vi "BMcalculate_v1_2.vi"() -> ()   [LabVIEW 2014]
uses:
  <vilib>/Analysis/coordinate.llb/2D Cartesian Coordinate Rotation (Array).vi
  <vilib>/Analysis/baseanly.llb/Mean (DBL).vi
  <vilib>/Utility/file.llb/Read From Spreadsheet File (string).vi
  <vilib>/Utility/file.llb/Write To Spreadsheet File (DBL).vi
  <vilib>/Analysis/NI_AALBase.lvlib
  <vilib>/Analysis/NI_AALPro.lvlib
panel:
  in  "Menu Ring":u16(ring) items=["No highlight", "Highlight"]
  out "created path 2":path
  out "created path":path
  in  "Save Time-trace":bool
  in  "nm/pixel":dbl=72.5 format="%#_13g"
  in  "Folder path":path
  in  "?":bool
  in  "~":dbl=1.15 format="%#_13g"
  in  "x/y for all":dbl=0.85 format="%#_13g"
  out "filename":string
  in  "Mode":u16(ring)=2 items=["Median_fix window", "Average_fix window", "Median_slide window", "Average_slide window"]
  in  "change to vertical ?":bool
  in  "?":enum32{"slide by slide", "delay"}(tab)=enum."delay"
  in  "?":bool
  in  "seconds to wait":u32
  in  "?":dbl=7.963 format="%#_13g"
  in  "?":dbl=48.61 format="%#_13g"
  in  "Save BM":bool
  in  "?":bool=TRUE
  in  "Save X-Y plot":bool
  in  "less than":dbl=0.2 format="%#_13g"
  in  "?":bool
  in  "?":bool
  in  "?":bool=TRUE
  in  "?":T1(tab)
  out "Filenames":string[](array[string])
  out "useful AOIs":i32[](array[numeric])
  out "# of AOI":i32[](array[numeric])
  out "% of useful AOIs":dbl
  out "tt # of AOIs":i32
  out "# of Frames":dbl[](array[numeric])
  out "tt # 0f useful AOIs":i32
  out "?":T2(graph)
  out "size(s)":i32
  out "X-Y plot":cluster{dbl[], dbl[]}(graph)
  out "Xstd":dbl
  out "ystd":dbl[](array[numeric])
  out "X":dbl format="%0.2f"
  out "Y":dbl format="%0.2f"
  out "?":T2(graph)
  out "tt # of useful AOIs":i32
  out "xstd":dbl[](array[numeric])
  out "# of AOI":i32
  out "y 2":dbl[](array[numeric])
  out "# of frames":dbl
  out "y":dbl[][](array[numeric])
  out "x":dbl[][](array[numeric])
  out "y":dbl[](array[numeric])
  out "x":dbl[](array[numeric])
  out "y":dbl[](array[numeric])
  out "x":dbl[](array[numeric])
  out "number":dbl[][](array[numeric])
  out "all rows":string[][](array[string])
  out "Useful aoi number":string[][](array[string])
  in  "Tab Control":enum32{"Highlight", "No Highlight"}(tab)=enum."No Highlight"
  out "Time trace HL":T3(graph)
  in  "Highlight":dbl=30.0
  in  "±":dbl=30.0
  out "aoi":string
  out "max-min":dbl
  out "Time trace":T3(graph)
  out "max-min":dbl
  out "aoi":string
  # "Critiria"
  # "±"
  # "23.776±6.613 nm"
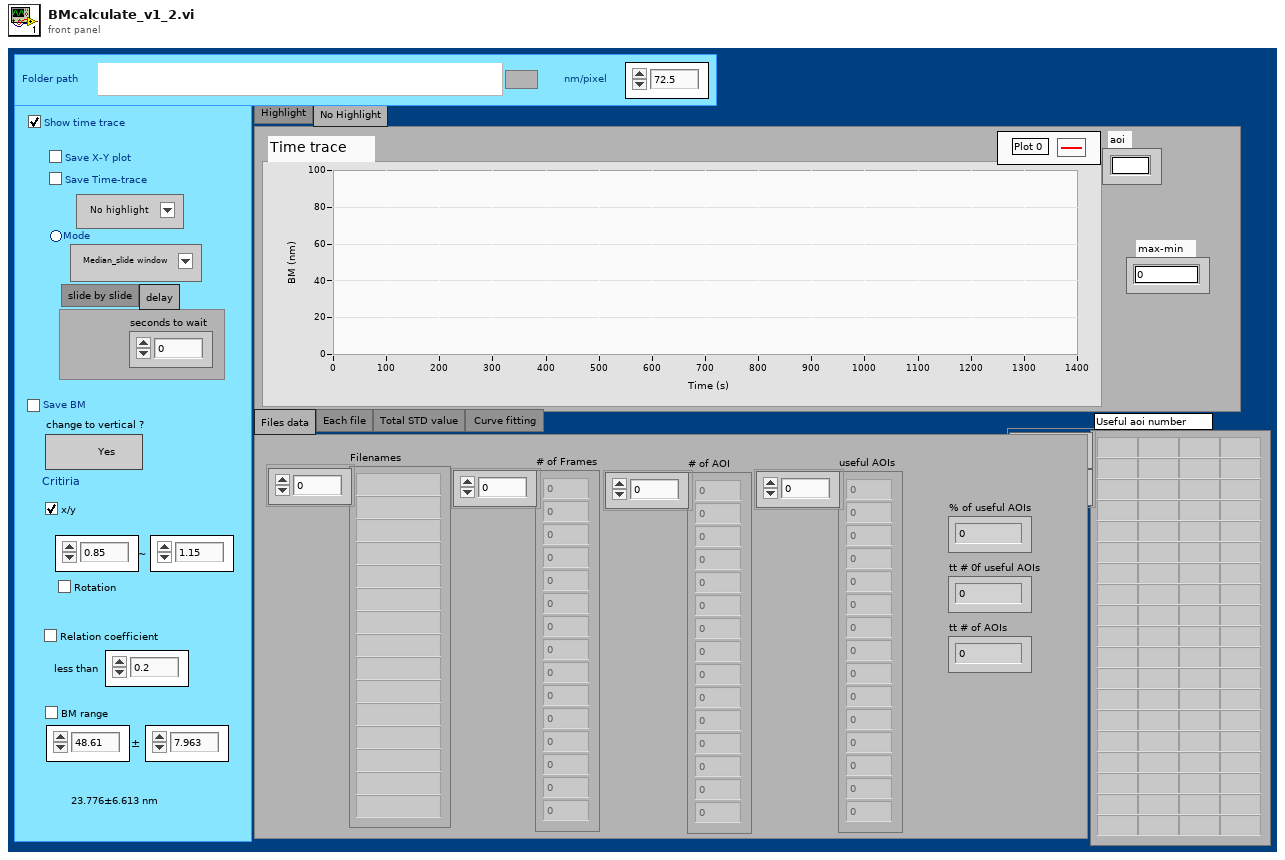
[diagram p1: front panel]
types:
  T1 = enum32{"Files data", "Each file", "Total STD value", "Curve fitting "}
  T2 = cluster{"X Values":dbl[], "Histogram: h(x)":i32[]}
  T3 = cluster{"Filtered X":dbl[], "Filtered X":dbl[]}[]
  T4 = typedef "imagedata.ctl" = cluster{"image type":i32, "image depth":i32, "image":u8[], "mask":u8[], "colors":u32[], "Rectangle":cluster{"left":i16, "top":i16, "right":i16, "bottom":i16}}
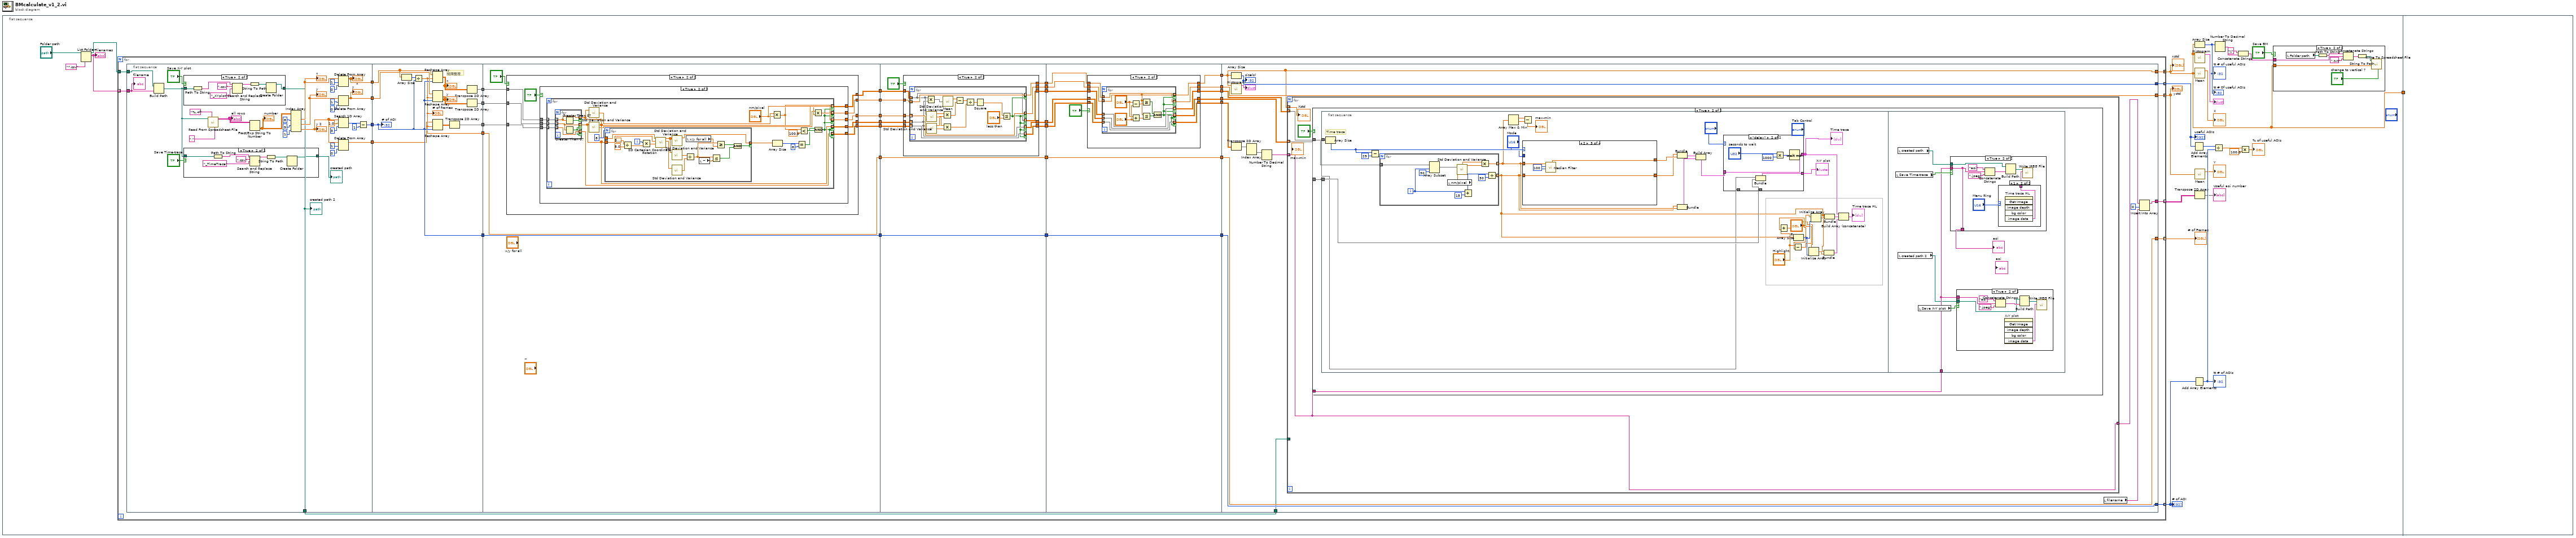
[diagram p0: block diagram]
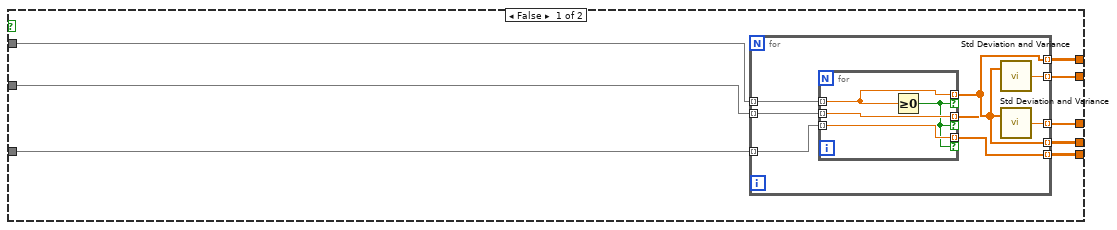
[diagram p5: hidden frame]
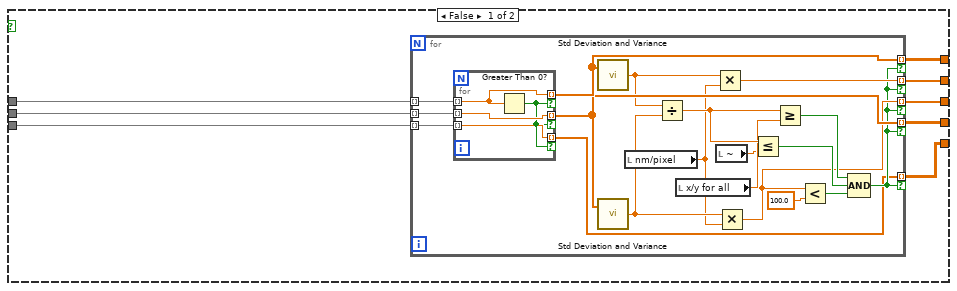
[diagram p6: hidden frame]
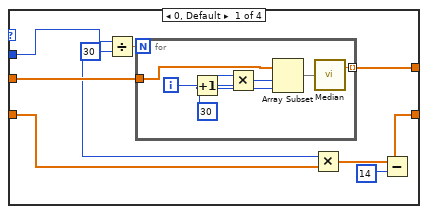
[diagram p10: hidden frame]
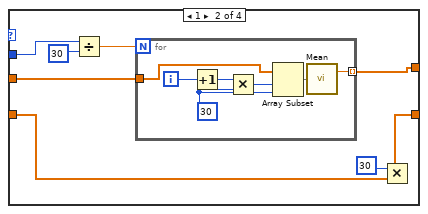
[diagram p11: hidden frame]
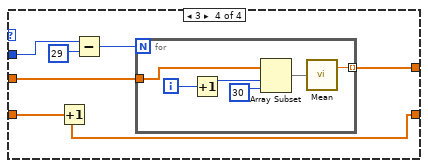
[diagram p12: hidden frame]
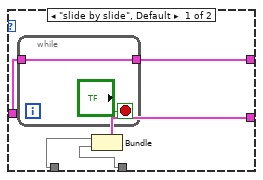
[diagram p13: hidden frame]
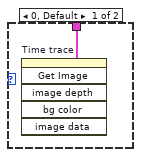
[diagram p16: hidden frame]
diagram:
  n1 = flat-sequence {
    tunnel: [w2] -> w1
    tunnel: w1 -> [_]
    frame #0 {
      n2 = List Folder(path="Folder path", pattern="*.csv") -> (path out=w24:path, filenames=w23:string[])  [unwired: 2 in, 2 out]
      "Filenames" <- w23
      n3 = for {
        tunnel: w24 -> [w37]
        tunnel: w23 -> [w72] mode=indexing
        tunnel: [w71] -> w2 mode=concatenating
        tunnel: [w70] -> w21 mode=indexing
        tunnel: [w69] -> w20 mode=indexing
        tunnel: [w68] -> w12 mode=concatenating
        tunnel: [w67] -> w13 mode=indexing
        tunnel: [w34] -> w4 mode=indexing
        n4 = flat-sequence {
          tunnel: [w92] -> w66
          tunnel: [w91] -> w65
          tunnel: [w85] -> w64
          tunnel: w37 -> [w80]
          tunnel: w72 -> [w76]
          tunnel: [w81] -> w41
          tunnel: [w79] -> w35
          tunnel: w66 -> [w128]
          tunnel: w65 -> [w127]
          tunnel: w64 -> [w124]
          tunnel: [w123] -> w63
          tunnel: [w124] -> w62
          tunnel: [w126] -> w61
          tunnel: [w125] -> w60
          tunnel: w41 -> [w122]
          tunnel: [w120] -> w40
          tunnel: w63 -> [w142]
          tunnel: w62 -> [w141]
          tunnel: w61 -> [w140]
          tunnel: w60 -> [w139]
          tunnel: [w141] -> w53
          tunnel: [w142] -> w51
          tunnel: [w137] -> w49
          tunnel: [w136] -> w47
          tunnel: [w135] -> w45
          tunnel: [w134] -> w43
          tunnel: w40 -> [w132]
          tunnel: [w133] -> w39
          tunnel: w53 -> [w265]
          tunnel: [w265] -> w52
          tunnel: w51 -> [w264]
          tunnel: [w264] -> w50
          tunnel: w49 -> [w260]
          tunnel: [w255] -> w48
          tunnel: w47 -> [w263]
          tunnel: [w258] -> w46
          tunnel: w45 -> [w262]
          tunnel: [w257] -> w44
          tunnel: w43 -> [w261]
          tunnel: [w256] -> w42
          tunnel: w39 -> [w254]
          tunnel: [w253] -> w38
          tunnel: w52 -> [w311]
          tunnel: w50 -> [w310]
          tunnel: w48 -> [w305]
          tunnel: [w311] -> w59
          tunnel: [w310] -> w58
          tunnel: [w304] -> w57
          tunnel: [w308] -> w56
          tunnel: w46 -> [w309]
          tunnel: [w306] -> w55
          tunnel: w44 -> [w307]
          tunnel: [w299] -> w54
          tunnel: w42 -> [w300]
          tunnel: w38 -> [w302]
          tunnel: [w301] -> w36
          tunnel: [w355] -> w68
          tunnel: [w356] -> w67
          tunnel: [w357] -> w69
          tunnel: [w351] -> w70
          tunnel: [w345] -> w71
          tunnel: w59 -> [w357]
          tunnel: w58 -> [w356]
          tunnel: w57 -> [w355]
          tunnel: w56 -> [w354]
          tunnel: w55 -> [w353]
          tunnel: w54 -> [w345]
          tunnel: w36 -> [w350]
          tunnel: w35 -> [w346]
          tunnel: [w341] -> w34
          frame #0 {
            n5 = Build Path(base path=w80, name or relative path=w76) -> (appended path=w74:path)
            n6 = case shown="True" "Save X-Y plot" {
              tunnel: w74 -> [w112 w119]
              tunnel: [w112 w113] -> w79
              frame False {
              }
              frame True {
                n7 = Path To String(path=w119) -> (string=w118:string)
                n8 = Search and Replace String(input string=w118, search string=".csv", replace string="_XYplot" ("replace string (\"\")")) -> (result string=w115:string)  [unwired: 5 in, 3 out]
                n9 = String To Path(string=w115) -> (path=w114:path)
                n10 = Create Folder(path (use dialog)=w114) -> (created path=w113:path)  [unwired: 2 in, 2 out]
              }
            }
            "created path 2" <- w79
            n11 = case shown="True" "Save Time-trace" {
              tunnel: w74 -> [w104 w111]
              tunnel: [w104 w105] -> w73
              frame False {
              }
              frame True {
                n12 = Path To String(path=w111) -> (string=w110:string)
                n13 = Search and Replace String(input string=w110, search string=".csv", replace string="_TimeTrace" ("replace string (\"\")")) -> (result string=w107:string)  [unwired: 5 in, 3 out]
                n14 = String To Path(string=w107) -> (path=w106:path)
                n15 = Create Folder(path (use dialog)=w106) -> (created path=w105:path)  [unwired: 2 in, 2 out]
              }
            }
            "created path" <- w73
            n16 = call-poly <vilib>:"Read From Spreadsheet File.vi"("delimiter (\\t)"="," ("delimiter (\\t)"), "format (%s)"="%.4f" ("format (%.3f)"), "file path (dialog if empty)"=w74) -> ("all rows"=w102:string[][])  [unwired: 4 in, 4 out]
            "all rows" <- w102
            n17 = Fract/Exp String To Number(string=w102) -> (number=w101:dbl[][])  [unwired: 3 in, 1 out]
            "number" <- w101
            n18 = Index Array(array=w101, index (col) #1=8 ("disabled index (col)"), index (col) #2=9 ("index (col)"), index (col) #3=1 ("index (col)")) -> (element #1=w93:dbl[], element #2=w94:dbl[], element #3=w82:dbl[])  [unwired: 3 in]
            "x" <- w93
            "y" <- w94
            "y 2" <- w82
            n19 = Delete From Array(array=w93, length=1, index=0) -> (array with subset deleted=w92:dbl[])  [unwired: 1 out]
            "x" <- w92
            n20 = Delete From Array(array=w94, length=1, index=0) -> (array with subset deleted=w91:dbl[])  [unwired: 1 out]
            "y" <- w91
            n21 = Search 1D Array(1D array=w82, element=1.0, start index (0)=3) -> (index of element=w87:i32)
            n22 = Delete From Array(array=w82, length=1, index=0) -> (array with subset deleted=w81:dbl[])  [unwired: 1 out]
            n23 = Subtract(x=w87, y=1) -> (x-y=w85:i32)
            "filename" <- w76
          }
          frame #1 {
            # "矩陣整理"
            n24 = Array Size(array=w128) -> (size(s)=w129:i32)
            n25 = Divide(x=w129, y=w124) -> (x/y=w123:dbl)
            "# of frames" <- w123
            n26 = Reshape Array(w128, w123, w124) -> (w130:dbl[][])
            "x" <- w130
            n27 = Reshape Array(w127, w123, w124) -> (w131:dbl[][])
            "y" <- w131
            n28 = Reshape Array(w122, w123, w124) -> (w121:dbl[][])
            n29 = Transpose 2D Array(2D array=w121) -> (transposed array=w120:dbl[][])
            n30 = Transpose 2D Array(2D array=w130) -> (transposed array=w126:dbl[][])
            n31 = Transpose 2D Array(2D array=w131) -> (transposed array=w125:dbl[][])
            "# of AOI" <- w124
          }
          frame #2 {
            n32 = case shown="True" "?" {
              tunnel: [w148 w171] -> w136
              tunnel: [w147 w170] -> w135
              tunnel: w140 -> [w150 w169]
              tunnel: w139 -> [w149 w168]
              tunnel: [w146 w167] -> w134
              tunnel: [w145 w166] -> w137
              tunnel: w132 -> [w144 w164]
              tunnel: [w143 w163] -> w133
              frame False {
                n33 = for {
                  tunnel: w150 -> [w158] mode=indexing
                  tunnel: w149 -> [w157] mode=indexing
                  tunnel: [w156] -> w148 mode=indexing
                  tunnel: [w155] -> w147 mode=indexing
                  tunnel: [w154] -> w146 mode=indexing
                  tunnel: [w153] -> w145 mode=indexing
                  tunnel: w144 -> [w152] mode=indexing
                  tunnel: [w151] -> w143 mode=indexing
                  n34 = for {
                    tunnel: w158 -> [w161] mode=indexing
                    tunnel: w157 -> [w162] mode=indexing
                    tunnel: [w161] -> w156 mode=indexing if=w159
                    tunnel: [w162] -> w155 mode=indexing if=w159
                    tunnel: w152 -> [w160] mode=indexing
                    tunnel: [w160] -> w151 mode=indexing if=w159
                    n35 = Greater Or Equal To 0?(x=w161) -> (x >= 0?=w159:bool)
                  }
                  n36 = call <vilib>:"Std Deviation and Variance.vi"("X"=w155) -> ("standard deviation"=w153:dbl)  [unwired: 1 in, 2 out]
                  n37 = call <vilib>:"Std Deviation and Variance.vi"("X"=w156) -> ("standard deviation"=w154:dbl)  [unwired: 1 in, 2 out]
                }
              }
              frame True {
                n38 = case shown="True" "?" {
                  tunnel: w168 -> [w178 w210]
                  tunnel: w169 -> [w179 w209]
                  tunnel: [w177 w208] -> w171
                  tunnel: [w176 w207] -> w170
                  tunnel: [w175 w206] -> w167
                  tunnel: [w174 w205] -> w166
                  tunnel: w164 -> [w173 w204]
                  tunnel: [w172 w203] -> w163
                  frame False {
                    n39 = for {
                      tunnel: w179 -> [w198] mode=indexing
                      tunnel: w178 -> [w197] mode=indexing
                      tunnel: [w196] -> w177 mode=indexing if=w183
                      tunnel: [w195] -> w176 mode=indexing if=w183
                      tunnel: [w184] -> w175 mode=indexing if=w183
                      tunnel: [w187] -> w174 mode=indexing if=w183
                      tunnel: [w181] -> w172 mode=indexing if=w183
                      tunnel: w173 -> [w182] mode=indexing
                      n40 = for {
                        tunnel: w198 -> [w201] mode=indexing
                        tunnel: w197 -> [w202] mode=indexing
                        tunnel: [w201] -> w196 mode=indexing if=w199
                        tunnel: [w202] -> w195 mode=indexing if=w199
                        tunnel: w182 -> [w200] mode=indexing
                        tunnel: [w200] -> w181 mode=indexing if=w199
                        n41 = Greater Than 0?(x=w201) -> (x > 0?=w199:bool)
                      }
                      n42 = call <vilib>:"Std Deviation and Variance.vi"("X"=w196) -> ("standard deviation"=w188:dbl)  [unwired: 1 in, 2 out]
                      n43 = call <vilib>:"Std Deviation and Variance.vi"("X"=w195) -> ("standard deviation"=w189:dbl)  [unwired: 1 in, 2 out]
                      n44 = local read "nm/pixel"() -> (w180:dbl)
                      n45 = Divide(x=w188, y=w189) -> (x/y=w194:dbl)
                      n46 = local read "x/y for all"() -> (w193:dbl)
                      n47 = Multiply(x=w188, y=w180) -> (x*y=w187:dbl)
                      n48 = local read "~"() -> (w192:dbl)
                      n49 = Multiply(x=w189, y=w180) -> (x*y=w184:dbl)
                      n50 = Less Or Equal?(x=w194, y=w192) -> (x <= y?=w190:bool)
                      n51 = Greater Or Equal?(x=w194, y=w193) -> (x >= y?=w191:bool)
                      n52 = Less?(x=w184, y=100.0) -> (x < y?=w185:bool)
                      n53 = Compound Arithmetic op=AND(w191, w190, w185) -> (w183:bool)
                    }
                  }
                  frame True {
                    n54 = for {
                      tunnel: w209 -> [w229] mode=indexing
                      tunnel: w210 -> [w228] mode=indexing
                      tunnel: [w214] -> w206 mode=indexing if=w213
                      tunnel: [w221] -> w207 mode=indexing if=w213
                      tunnel: [w222] -> w208 mode=indexing if=w213
                      tunnel: [w219] -> w205 mode=indexing if=w213
                      tunnel: [w211] -> w203 mode=indexing if=w213
                      tunnel: w204 -> [w212] mode=indexing
                      n55 = for {
                        tunnel: [w232] -> w221 mode=indexing if=w230
                        tunnel: [w233] -> w222 mode=indexing if=w234
                        tunnel: w229 -> [w233] mode=indexing
                        tunnel: w228 -> [w232] mode=indexing
                        tunnel: [w231] -> w211 mode=indexing if=w230
                        tunnel: w212 -> [w231] mode=indexing
                        n56 = Greater Than 0?(x=w233) -> (x > 0?=w234:bool)
                        n57 = Greater Than 0?(x=w232) -> (x > 0?=w230:bool)
                      }
                      n58 = call <vilib>:"Std Deviation and Variance.vi"("X"=w222) -> ("standard deviation"=w223:dbl)  [unwired: 1 in, 2 out]
                      n59 = call <vilib>:"Std Deviation and Variance.vi"("X"=w221) -> ("standard deviation"=w220:dbl)  [unwired: 1 in, 2 out]
                      n60 = for {
                        N: 8 -> [_]
                        tunnel: w222 -> [w247]
                        tunnel: w221 -> [w246]
                        tunnel: [w238] -> w224 mode=indexing if=w237
                        i -> [w248]
                        n61 = Divide(x=3.141592653589793, y=8.0) -> (x/y=w251:dbl)
                        n62 = Multiply(x=w248, y=w251) -> (x*y=w249:dbl)
                        n63 = call-poly <vilib>:"2D Cartesian Coordinate Rotation.vi"("theta"=w249, "Y"=w246, "X"=w247) -> ("Y Out"=w239:dbl[], "X Out"=w240:dbl[])  [unwired: 6 in, 1 out]
                        n64 = call <vilib>:"Std Deviation and Variance.vi"("X"=w240) -> ("mean"=w238:dbl)  [unwired: 1 in, 2 out]
                        n65 = call <vilib>:"Std Deviation and Variance.vi"("X"=w240) -> ("standard deviation"=w245:dbl)  [unwired: 1 in, 2 out]
                        n66 = call <vilib>:"Std Deviation and Variance.vi"("X"=w239) -> ("standard deviation"=w244:dbl)  [unwired: 1 in, 2 out]
                        n67 = Divide(x=w245, y=w244) -> (x/y=w243:dbl)
                        n68 = local read "x/y for all"() -> (w236:dbl)
                        n69 = local read "~"() -> (w235:dbl)
                        n70 = Less Or Equal?(x=w243, y=w235) -> (x <= y?=w241:bool)
                        n71 = Greater Or Equal?(x=w243, y=w236) -> (x >= y?=w242:bool)
                        n72 = Compound Arithmetic op=AND(w242, w241) -> (w237:bool)
                      }
                      n73 = Multiply(x=w223, y="nm/pixel") -> (x*y=w214:dbl)
                      n74 = Array Size(array=w224) -> (size(s)=w226:i32)
                      n75 = Equal?(x=w226, y=8) -> (x = y?=w215:bool)
                      n76 = Less?(x=w214, y=100.0) -> (x < y?=w216:bool)
                      n77 = Multiply(x=w220, y="nm/pixel") -> (x*y=w219:dbl)
                      n78 = Compound Arithmetic op=AND(w215, w216) -> (w213:bool)
                    }
                  }
                }
              }
            }
          }
          frame #3 {
            n79 = case shown="True" "?" {
              tunnel: w263 -> [w270 w280]
              tunnel: w262 -> [w269 w279]
              tunnel: w261 -> [w268 w276]
              tunnel: w260 -> [w267 w274]
              tunnel: [w270 w278] -> w258
              tunnel: [w269 w277] -> w257
              tunnel: [w268 w275] -> w256
              tunnel: [w267 w273] -> w255
              tunnel: w254 -> [w266 w272]
              tunnel: [w266 w271] -> w253
              frame False {
              }
              frame True {
                n80 = for {
                  tunnel: w280 -> [w286] mode=indexing
                  tunnel: w279 -> [w285] mode=indexing
                  tunnel: [w286] -> w278 mode=indexing if=w281
                  tunnel: [w285] -> w277 mode=indexing if=w281
                  tunnel: [w293] -> w275 mode=indexing if=w281
                  tunnel: w276 -> [w293] mode=indexing
                  tunnel: w274 -> [w292] mode=indexing
                  tunnel: [w292] -> w273 mode=indexing if=w281
                  tunnel: [w282] -> w271 mode=indexing if=w281
                  tunnel: w272 -> [w282] mode=indexing
                  n81 = Multiply(x=w286, y=w285) -> (x*y=w284:dbl[])
                  n82 = call <vilib>:"Std Deviation and Variance.vi"("X"=w286) -> ("mean"=w289:dbl, "standard deviation"=w291:dbl)  [unwired: 1 in, 1 out]
                  n83 = call <vilib>:"Std Deviation and Variance.vi"("X"=w285) -> ("mean"=w288:dbl, "standard deviation"=w290:dbl)  [unwired: 1 in, 1 out]
                  n84 = Multiply(x=w289, y=w288) -> (x*y=w287:dbl)
                  n85 = Multiply(x=w291, y=w290) -> (x*y=w294:dbl)
                  n86 = call-poly <vilib>:"Mean.vi"("X"=w284) -> ("mean"=w283:dbl)  [unwired: 1 out]
                  n87 = Subtract(x=w283, y=w287) -> (x-y=w295:dbl)
                  n88 = Divide(x=w295, y=w294) -> (x/y=w296:dbl)
                  n89 = Square(x=w296) -> (x^2=w297:dbl)
                  n90 = Less Or Equal?(x=w297, y="less than") -> (x <= y?=w281:bool)
                }
              }
            }
          }
          frame #4 {
            n91 = case shown="True" "?" {
              tunnel: [w317 w327] -> w308
              tunnel: w309 -> [w317 w328]
              tunnel: w307 -> [w316 w326]
              tunnel: [w316 w325] -> w306
              tunnel: w300 -> [w315 w324]
              tunnel: [w315 w323] -> w299
              tunnel: w305 -> [w314 w322]
              tunnel: [w314 w321] -> w304
              tunnel: w302 -> [w313 w320]
              tunnel: [w312 w319] -> w301
              frame False {
                n92 = for {
                  tunnel: w313 -> [w318] mode=indexing
                  tunnel: [w318] -> w312 mode=indexing
                }
              }
              frame True {
                n93 = for {
                  tunnel: [w340] -> w327 mode=indexing if=w335
                  tunnel: w328 -> [w340] mode=indexing
                  tunnel: [w339] -> w325 mode=indexing if=w335
                  tunnel: w326 -> [w339] mode=indexing
                  tunnel: [w329] -> w323 mode=indexing if=w335
                  tunnel: w324 -> [w329] mode=indexing
                  tunnel: w322 -> [w334] mode=indexing
                  tunnel: [w334] -> w321 mode=indexing if=w335
                  tunnel: [w336] -> w319 mode=indexing if=w335
                  tunnel: w320 -> [w336] mode=indexing
                  n94 = Subtract(x="?", y="?") -> (x-y=w331:dbl)
                  n95 = Add(x="?", y="?") -> (x+y=w330:dbl)
                  n96 = Greater Or Equal?(x=w329, y=w331) -> (x >= y?=w338:bool)
                  n97 = Less Or Equal?(x=w329, y=w330) -> (x <= y?=w337:bool)
                  n98 = Compound Arithmetic op=AND(w338, w337) -> (w335:bool)
                }
              }
            }
          }
          frame #5 {
            n99 = Array Size(array=w345) -> (size(s)=w351:i32)
            "size(s)" <- w351
            n100 = call <vilib>:"Histogram.vi"("X"=w345) -> ("Histogram Graph"=→"?":T2)  [unwired: 7 in, 3 out]
            n101 = Transpose 2D Array(2D array=w350) -> (transposed array=w349:dbl[][])
            n102 = Index Array(array=w349) -> (element=w348:dbl[])  [unwired: 2 in]
            n103 = Number To Decimal String(number=w348) -> (decimal integer string=w347:string[])  [unwired: 1 in]
            n104 = for {
              tunnel: w354 -> [w361] mode=indexing
              tunnel: w353 -> [w362] mode=indexing
              tunnel: w347 -> [w358] mode=indexing
              tunnel: w346 -> [_]
              tunnel: w345 -> [w359] mode=indexing
              tunnel: [w358] -> w342 mode=indexing
              n105 = case shown="True" "?" {
                tunnel: w362 -> [_ w365]
                tunnel: w361 -> [_ w364]
                tunnel: w358 -> [_ w363]
                frame False {
                }
                frame True {
                  n106 = flat-sequence {
                    tunnel: w365 -> [w378]
                    tunnel: w364 -> [w377]
                    tunnel: w363 -> [w471]
                    frame #0 {
                      # "Time trace"
                      n107 = Array Size(array=w377) -> (size(s)=w384:i32)
                      n108 = Subtract(x=w384, y=29) -> (x-y=w393:i32)
                      n109 = for {
                        N: w393 -> [_]
                        tunnel: w377 -> [w467]
                        tunnel: [w458] -> w375 mode=indexing
                        tunnel: [w460] -> w371 mode=indexing
                        i -> [w459]
                        n110 = Array Subset(array=w467, index=w459, length=30) -> (w465:dbl[])
                        n111 = local read "nm/pixel"() -> (w457:dbl)
                        n112 = call <vilib>:"Std Deviation and Variance.vi"("X"=w465) -> ("standard deviation"=w464:dbl)  [unwired: 1 in, 2 out]
                        n113 = Add(x=w459, y=15) -> (x+y=w462:i32)
                        n114 = Multiply(x=w464, y=w457) -> (x*y=w458:dbl)
                        n115 = Divide(x=w462, y=30) -> (x/y=w460:dbl)
                      }
                      n116 = Array Max & Min(array=w375) -> (max value=w390:dbl, min value=w389:dbl)  [unwired: 2 out]
                      n117 = case shown="2" "Mode" {
                        tunnel: [w402 w417 w427 w435] -> w392
                        tunnel: w375 -> [w403 w418 w428 w436]
                        tunnel: w384 -> [w401 w416 _ w434]
                        tunnel: w371 -> [w399 w412 w426 w431]
                        tunnel: [w396 w411 w426 w430] -> w376
                        frame 0, Default {
                          w397 = 30 ("y")
                          n118 = Divide(x=w401, y=w397) -> (x/y=w400:dbl)
                          n119 = for {
                            N: w400 -> [_]
                            tunnel: w403 -> [w410]
                            tunnel: [w406] -> w402 mode=indexing
                            i -> [w409]
                            w404 = 30 ("length")
                            n120 = Increment(x=w409) -> (x+1=w408:i32)
                            n121 = Multiply(x=w404, y=w408) -> (x*y=w405:i32)
                            n122 = Array Subset(array=w410, index=w405, length=w404) -> (w407:dbl[])
                            n123 = call <vilib>:"Median.vi"("X"=w407) -> ("median"=w406:dbl)  [unwired: 1 out]
                          }
                          n124 = Multiply(x=w397, y=w399) -> (x*y=w398:dbl[])
                          n125 = Subtract(x=w398, y=14) -> (x-y=w396:dbl[])
                        }
                        frame 1 {
                          n126 = Divide(x=w416, y=30) -> (x/y=w414:dbl)
                          n127 = for {
                            N: w414 -> [_]
                            tunnel: w418 -> [w425]
                            tunnel: [w422] -> w417 mode=indexing
                            i -> [w424]
                            w419 = 30 ("length")
                            n128 = Increment(x=w424) -> (x+1=w420:i32)
                            n129 = Multiply(x=w420, y=w419) -> (x*y=w421:i32)
                            n130 = Array Subset(array=w425, index=w421, length=w419) -> (w423:dbl[])
                            n131 = call-poly <vilib>:"Mean.vi"("X"=w423) -> ("mean"=w422:dbl)  [unwired: 1 out]
                          }
                          n132 = Multiply(x=30 ("length"), y=w412) -> (x*y=w411:dbl[])
                        }
                        frame 2 {
                          w429 = 100 ("left rank")
                          n133 = call <vilib>:"Median Filter.vi"("right rank"=w429, "left rank"=w429, "X"=w428) -> ("Filtered X"=w427:dbl[])  [unwired: 7 in, 1 out]
                        }
                        frame 3 {
                          n134 = Increment(x=w431) -> (x+1=w430:dbl[])
                          n135 = Subtract(x=w434, y=29) -> (x-y=w432:i32)
                          n136 = for {
                            N: w432 -> [_]
                            tunnel: w436 -> [w442]
                            tunnel: [w439] -> w435 mode=indexing
                            i -> [w441]
                            n137 = Increment(x=w441) -> (x+1=w437:i32)
                            n138 = Array Subset(array=w442, index=w437, length=30) -> (w440:dbl[])
                            n139 = call-poly <vilib>:"Mean.vi"("X"=w440) -> ("mean"=w439:dbl)  [unwired: 1 out]
                          }
                        }
                      }
                      n140 = Subtract(x=w390, y=w389) -> (x-y=→"max-min":dbl)
                      n141 = Bundle(w376, "Filtered X"=w392) -> (w391:cluster{dbl[], "Filtered X":dbl[]})  [unwired: 1 in]
                      n142 = Bundle(w371, w375) -> (w383:cluster{dbl[], dbl[]})  [unwired: 1 in]
                      n143 = Build Array(w391, w383) -> (w387:cluster{dbl[], "Filtered X":dbl[]}[])
                      n144 = case shown="\"delay\"" "?" {
                        tunnel: w387 -> [w447 w456]
                        tunnel: [w446 w456] -> w379
                        tunnel: w377 -> [w445 w452]
                        tunnel: w378 -> [w444 w451]
                        tunnel: [w443 w450] -> w382
                        frame "slide by slide", Default {
                          n145 = while {
                            tunnel: w447 -> [w448]
                            tunnel: [w448] -> w446
                            stop <- "?" stop-if-true
                          }
                          n146 = Bundle(w445, w444) -> (w443:cluster{dbl[], dbl[]})  [unwired: 1 in]
                        }
                        frame "delay" {
                          n147 = Bundle(w452, w451) -> (w450:cluster{dbl[], dbl[]})  [unwired: 1 in]
                          n148 = Multiply(x="seconds to wait", y=u32 1000) -> (x*y=w454:u32)
                          n149 = Wait (ms)(milliseconds to wait=w454) -> ()  [unwired: 1 out]
                        }
                      }
                      "Time trace" <- w379
                      "X-Y plot" <- w382
                      n150 = Add(x="Highlight", y="±") -> (x+y=w366:dbl)
                      n151 = Subtract(x="Highlight", y="±") -> (x-y=w367:dbl)
                      n152 = Array Size(array=w371) -> (size(s)=w373:i32)
                      n153 = Initialize Array(w366, w373) -> (w372:dbl[])
                      n154 = Initialize Array(w367, w373) -> (w374:dbl[])
                      n155 = Bundle(w371, w372) -> (w370:cluster{dbl[], dbl[]})  [unwired: 1 in]
                      n156 = Bundle(w371, w374) -> (w381:cluster{dbl[], dbl[]})  [unwired: 1 in]
                      n157 = Build Array (concatenate)(w379, w381, w370) -> (→"Time trace HL":cluster{dbl[], "Filtered X":dbl[]}[])
                    }
                    frame #1 {
                      n158 = local read "Save Time-trace"() -> (w472:bool)
                      n159 = local read "created path"() -> (w470:path)
                      n160 = local read "created path 2"() -> (w468:path)
                      n161 = local read "Save X-Y plot"() -> (w469:bool)
                      n162 = case shown="True" w472 {
                        tunnel: w471 -> [w481 w483]
                        tunnel: w470 -> [_ w487]
                        tunnel: [w481 w483] -> w473
                        frame False {
                        }
                        frame True {
                          n163 = Concatenate Strings("aoi" ("string"), w483, ".jpeg" ("string")) -> (w488:string)
                          n164 = case shown="1" "Menu Ring" {
                            tunnel: [w490 w491] -> w484
                            frame 0, Default {
                              n165 = invoke on="Time trace" class="XYGraph (strict)" method="Get Image"() -> ("image data"=w490:T4)  [unwired: 6 in, 5 out]
                            }
                            frame 1 {
                              n166 = invoke on="Time trace HL" class="XYGraph (strict)" method="Get Image"() -> ("image data"=w491:T4)  [unwired: 6 in, 5 out]
                            }
                          }
                          n167 = Build Path(base path=w487, name or relative path=w488) -> (appended path=w486:path)
                          n168 = call <vilib>:"Write JPEG File.vi"("image data"=w484, "path to JPEG file"=w486) -> ()  [unwired: 8 in, 2 out]
                        }
                      }
                      "aoi" <- w473
                      n169 = case shown="True" w469 {
                        tunnel: w471 -> [_ w480]
                        tunnel: w468 -> [_ w477]
                        frame False {
                        }
                        frame True {
                          n170 = Concatenate Strings("aoi" ("string"), w480, ".jpeg" ("string")) -> (w478:string)
                          n171 = invoke on="X-Y plot" class="XYGraph (strict)" method="Get Image"() -> ("image data"=w475:T4)  [unwired: 6 in, 5 out]
                          n172 = Build Path(base path=w477, name or relative path=w478) -> (appended path=w476:path)
                          n173 = call <vilib>:"Write JPEG File.vi"("image data"=w475, "path to JPEG file"=w476) -> ()  [unwired: 8 in, 2 out]
                        }
                      }
                    }
                  }
                }
              }
              "Xstd" <- w359
            }
            n174 = local read "filename"() -> (w344:string)
            n175 = Insert Into Array(array=w342, index=0, new element=w344) -> (w341:string[])
          }
        }
      }
      "useful AOIs" <- w21
      "# of AOI" <- w20
      "ystd" <- w12
      "# of Frames" <- w13
      "xstd" <- w2
      n176 = Add Array Elements(numeric array=w21) -> (sum=w19:i32)
      n177 = Add Array Elements(numeric array=w20) -> (sum=w18:i32)
      "tt # of AOIs" <- w18
      n178 = Array Size(array=w2) -> (size(s)=w9:i32)
      "tt # 0f useful AOIs" <- w9
      "tt # of useful AOIs" <- w9
      n179 = call <vilib>:"Histogram.vi"("X"=w2) -> ("Histogram Graph"=→"?":T2)  [unwired: 7 in, 3 out]
      n180 = call-poly <vilib>:"Mean.vi"("X"=w2) -> ("mean"=→"X":dbl)  [unwired: 1 out]
      n181 = call-poly <vilib>:"Mean.vi"("X"=w12) -> ("mean"=→"Y":dbl)  [unwired: 1 out]
      n182 = Transpose 2D Array(2D array=w4) -> (transposed array=→"Useful aoi number":string[][])
      n183 = Divide(x=w19, y=w18) -> (x/y=w17:dbl)
      n184 = Number To Decimal String(number=w9) -> (decimal integer string=w7:string)  [unwired: 1 in]
      n185 = Concatenate Strings("\\" ("string"), w7) -> (w6:string)
      n186 = Multiply(x=w17, y=100.0) -> (x*y=→"% of useful AOIs":dbl)
      n187 = case shown="True" "Save BM" {
        tunnel: w2 -> [_ w33]
        tunnel: w6 -> [_ w27]
        frame False {
        }
        frame True {
          n188 = local read "Folder path"() -> (w32:path)
          n189 = Path To String(path=w32) -> (string=w31:string)
          n190 = Concatenate Strings(w31, w27, ".txt" ("string")) -> (w30:string)
          n191 = String To Path(string=w30) -> (path=w29:path)
          n192 = call-poly <vilib>:"Write To Spreadsheet File.vi"("transpose? (no:F)"="change to vertical ?", "1D data"=w33, "file path (dialog if empty)"=w29) -> ()  [unwired: 5 in, 1 out]
        }
      }
    }
    frame #1 {
    }
  }
